vi "Read Attributes Initialized.vi"(8 "error in (no error)":errorcluster, 11 "CS++Base in":refnum<class "CS++Base.lvclass">) -> (0 "error out":errorcluster, 2 "Attributes Initialized":bool, 3 "CS++Base out":refnum<class "CS++Base.lvclass">)   [LabVIEW 2013, in "CS++BaseClasses.lvlib" / "CS++Base.lvclass"]
doc: "True if the <b>Initialize Attributes.vi</B> was called else false."
uses:
  CS++Base.lvclass
  CS++Base.lvclass/CS++Base.ctl
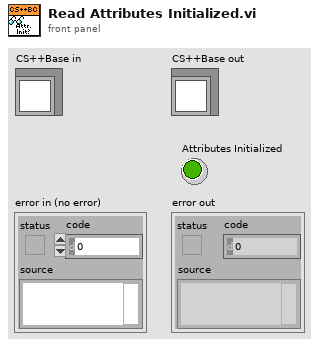
[diagram p1: front panel]
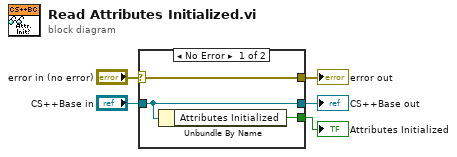
[diagram p0: block diagram]
diagram:
  n1 = case shown="No Error" "error in (no error)" {
    selector: "error in (no error)" -> [w8 w9]
    tunnel: [w8 w9] -> w4
    tunnel: [w7 w10] -> w2
    tunnel: "CS++Base in" -> [w7 w10]
    tunnel: [w6 _] -> w1
    frame No Error {
      n2 = Unbundle By Name(w7) -> ("Attributes Initialized"=w6:bool)
    }
    frame Error {
    }
  }
  "error out" <- w4
  "CS++Base out" <- w2
  "Attributes Initialized" <- w1
